vi "Select CDMA2000 Link Type.vi"(0 "VISA Resource Name":refnum<visa-resource-name>, 5 "Link Type (0: Forward)":enum16{"Forward", "Reverse"}(ring), 11 "error in (no error)":errorcluster {"code" format="%.0x"}) -> (4 "VISA Resource Name Out":refnum<visa-resource-name>, 15 "error out":errorcluster {"code" format="%.0x"})   [LabVIEW 2012, in "Agilent ESG Series.lvlib"]
doc: "This VI selects the CDMA2000 forward or reverse link channel setup.\n\nThis VI is valid only on instruments E44xxB with the 101 options or on instrument E4438C with option 401."
uses:
  <instrlib>/Agilent ESG Series/Agilent ESG Series.lvlib
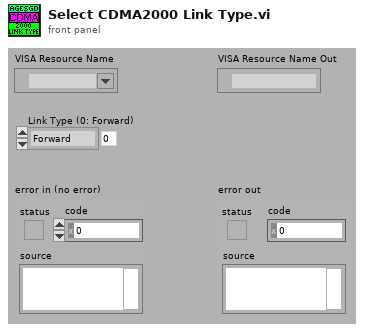
[diagram p1: front panel]
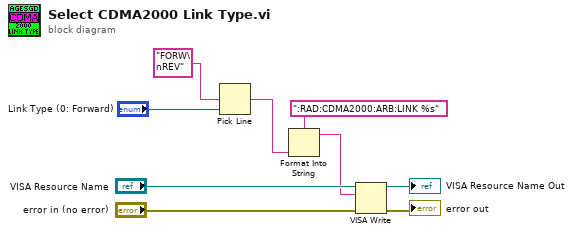
[diagram p0: block diagram]
diagram:
  n1 = Pick Line(multi-line string="FORW\nREV", line index="Link Type (0: Forward)") -> (output string=w3:string)  [unwired: 1 in]
  n2 = Format Into String(format string=":RAD:CDMA2000:ARB:LINK %s", w3) -> (resulting string=w2:string)  [unwired: 2 in, 1 out]
  n3 = VISA Write(VISA resource name="VISA Resource Name", write buffer=w2, error in (no error)="error in (no error)") -> (VISA resource name out=→"VISA Resource Name Out":refnum<visa-resource-name>, error out=→"error out":errorcluster)  [unwired: 1 out]
